vi "OLD_GUI_DO_NOT_USE-Capacitance.vi"() -> ()   [LabVIEW 2020]
uses:
  <vilib>/Utility/NIReport.llb/NI_report.lvclass
  <vilib>/Utility/NIReport.llb/Report Type.ctl
  <vilib>/addons/_office/_exclsub.llb/font.ctl
  <vilib>/addons/_office/excel.llb/Excel Easy Table (str).vi
  HP 4275A Address constant.vi
  HP 3457A Address constant.vi
  Keithley K2400 Address constant.vi
  <vilib>/Utility/NIReport.llb/NI_ReportGenerationCore.lvlib
  <vilib>/Utility/NIReport.llb/Excel/NI_Excel.lvclass
  <vilib>/addons/_office/NI_ReportGenerationToolkit.lvlib
panel:
  out "report out":refnum<class "NI_report.lvclass">
  out "error out":errorcluster
  in  "Filename":string
  in  "Test Mode":u16(ring) items=["Measure Capacitance", "Measure Series Impedance"]
  in  "function B\n(d or x/b:0)":i16(slide) scale=0.0..2.0 scale format="%.2f"
  in  "function A (c:1)":i16(slide)=1 scale=0.0..3.0 scale format="%.2f"
  out "Part Number to be Tested":u16
  in  "Number of Parts":i32
  in  "outside border":T1={"on/off"=FALSE, "weight"=2, "color"=0} {"weight" items=["xlHairline"=1, "xlMedium"=-4138, "xlThick"=4, "xlThin"=2]}
  in  "inside border":T1={"on/off"=FALSE, "weight"=2, "color"=0} {"weight" items=["xlHairline"=1, "xlMedium"=-4138, "xlThick"=4, "xlThin"=2]}
  in  "Next Part":bool
  in  "Max Voltage":dbl
  in  "Test Frequncy":string(combo)
  in  "Test System":string(combo)
  in  "Test Type":string(combo)
  in  "Date":string
  in  "Operator Name":string
  in  "Test Comments":string
  in  "Lot/Date Code":string
  in  "Lot Number":string
  in  "Request ID Number":string
  in  "Part Number":string
  in  "window state (normal)":T2(ring)=enum."normal"
  in  "FET Test Configuration":u16(ring) items=["CISS: VDS is variable, VGS=0V BLACK Jacks", "COSS: VDS is variable, a BLACK Jacks", "CRSS: VDS is variable, VGS=0V BLACK Jacks", "CISS: VDS is variable, VGS=0V RED Jacks", "COSS: VDS is variable, VGS=0V RED Jacks", "CRSS: VDS is variable, VGS=0V RED Jacks", "CIES: VDS is variable, VGS=0V Black Jacks", "CIES: VGS is variable, VDS=0V Red Jacks", "COES: VDS is variable, VGS=0V Black Jacks", "COES: VGS is variable, VDS=0V Red Jacks", "CRES: VDS is variable, VGS=0V Black Jacks", "CRES: VGS is variable, VDS=0V Red Jacks", "Special"]
  in  "Device":u16(ring) items=["Diode", "Transistor", "BRT", "MOSFET", "MOSFET with Gate Resistor", "JFET", "SSOVP", "SIDAC", "Bidirectional Zener", "SRC or TRIAC", "Darlington Transistor", "MicroIntegration", "IGBT", "IGBT with Gate Resistor", "Other"]
  in  "Transistor Test Configuration":u16(ring) items=["Cobo (Cob)", "Cibo (Cib)", "Coe", "Ccb (Cre)", "Ceb (Crc)", "Crb (Cce)", "Special"]
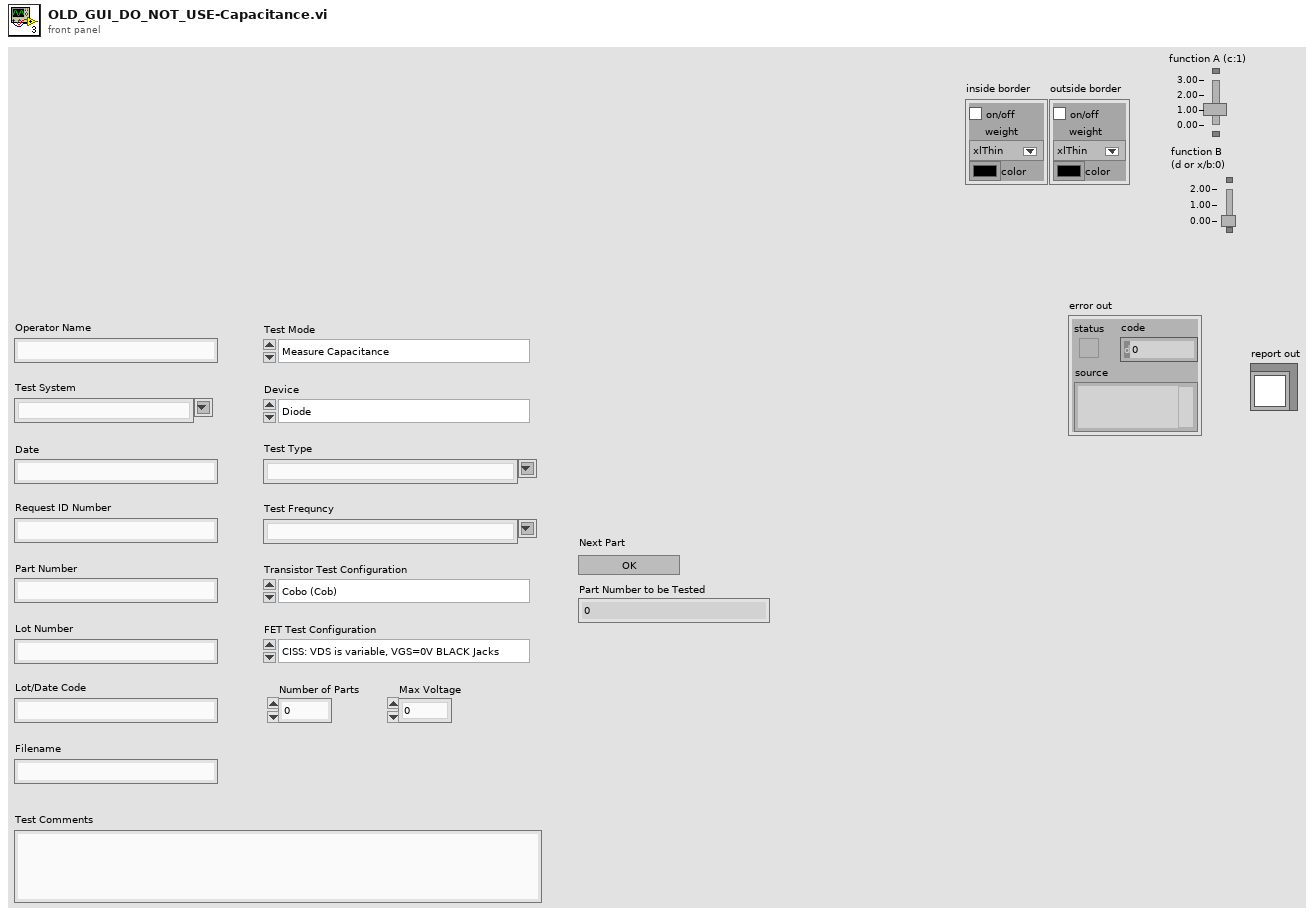
[diagram p1: front panel]
types:
  T1 = cluster{"on/off":bool, "weight":i32, "color":u32}
  T2 = enum16{"maximized", "minimized", "normal", "no change"}
  T3 = typedef "NI_ReportGenerationToolkit.lvlib/font.ctl" = cluster{"font name":string, "font size":dbl, "bold":u16, "italic":u16, "underline":u16, "strike through":u16, "font color":u32}
  T4 = typedef "NI_ReportGenerationCore.lvlib/Report Type.ctl" = enum16{"HTML", "Word", "Excel"}
  T5 = typedef "Control 1.ctl" = string
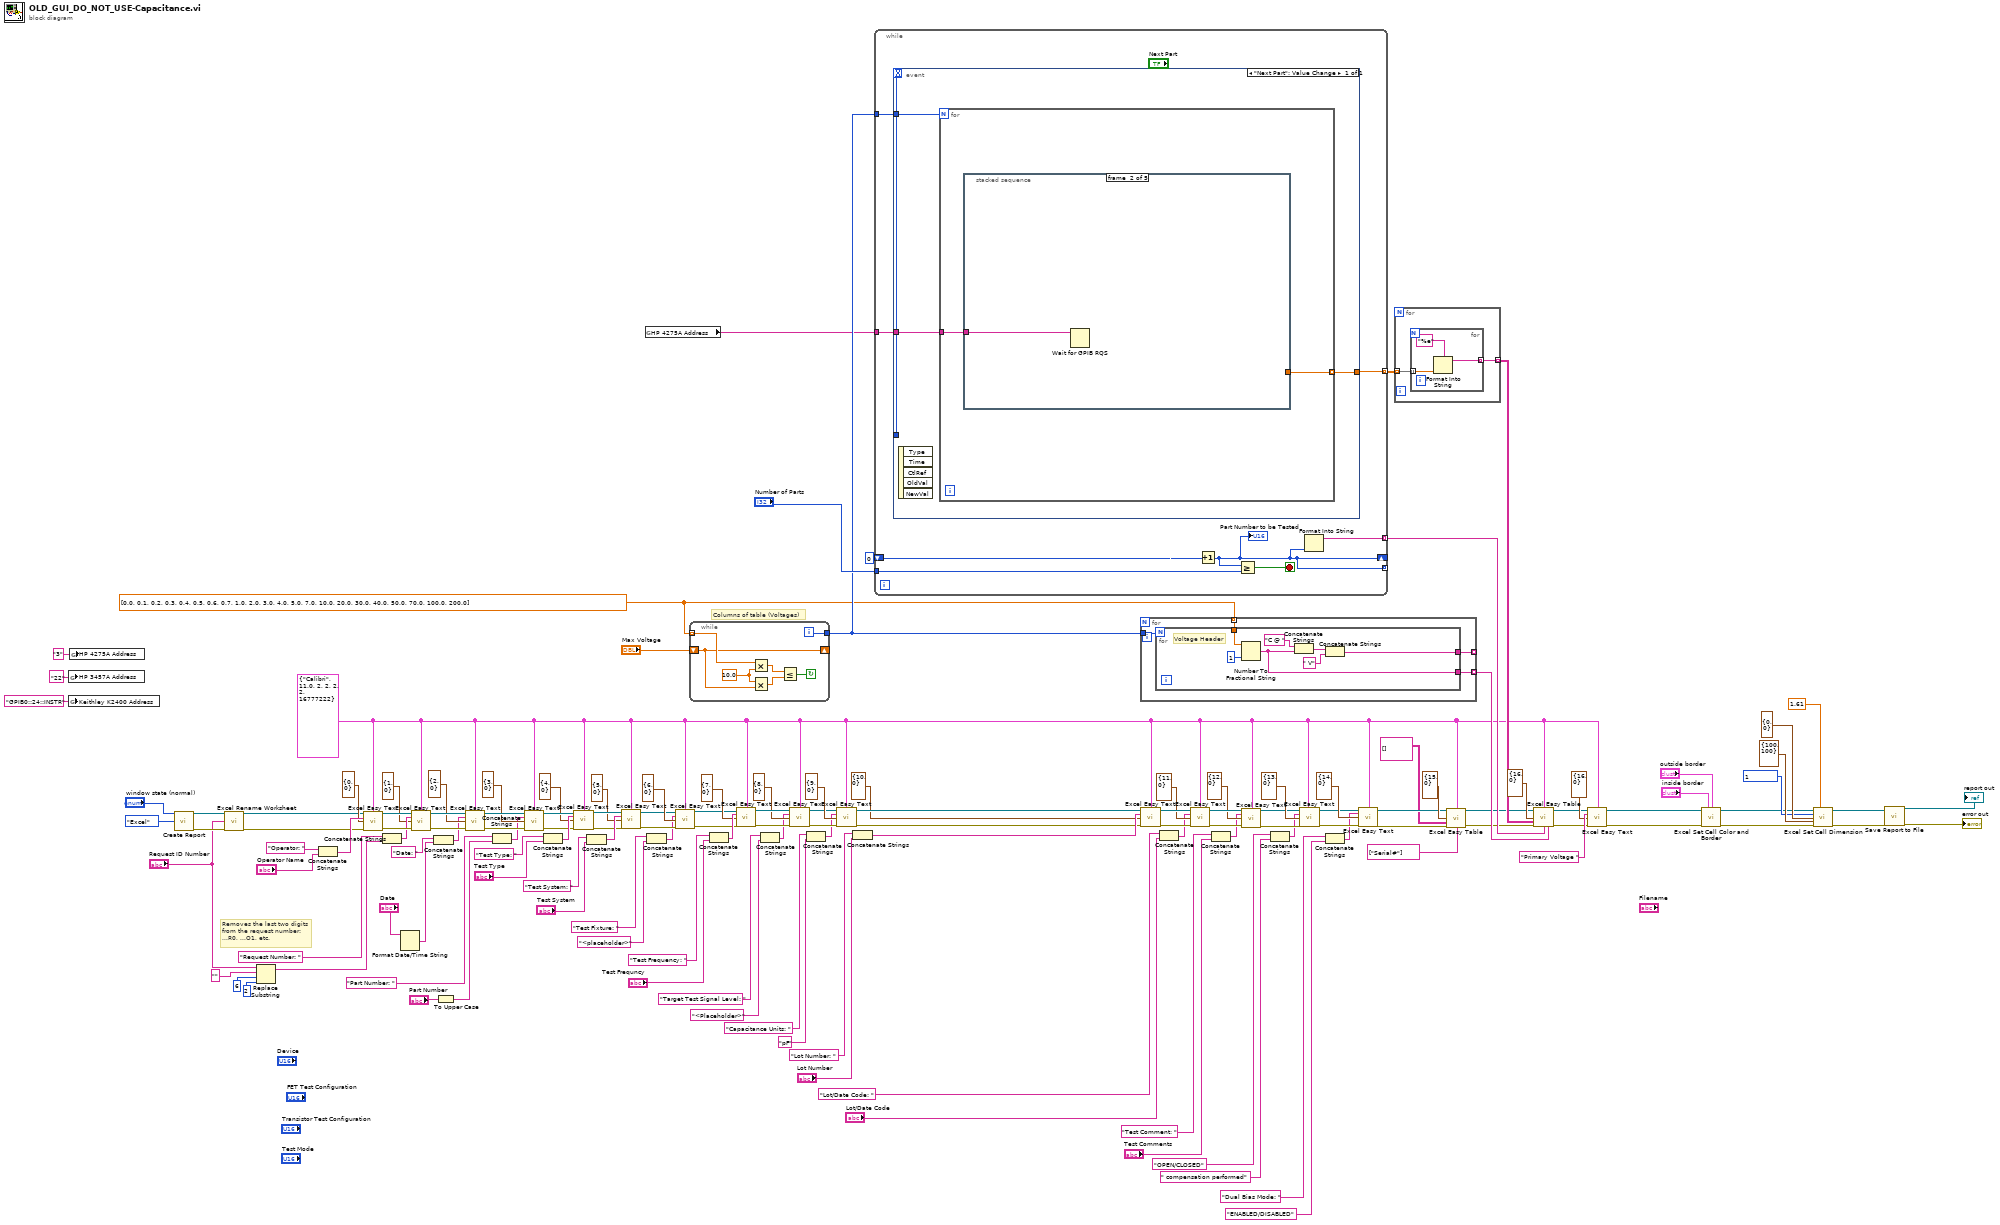
[diagram p0: block diagram]
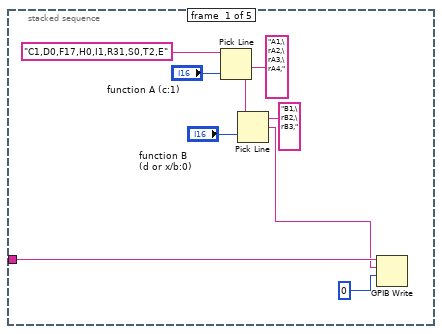
[diagram p2: hidden frame]
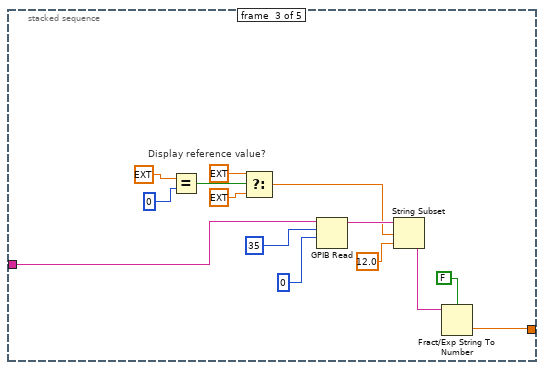
[diagram p3: hidden frame]
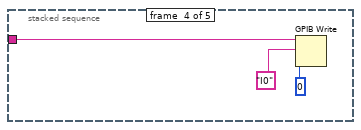
[diagram p4: hidden frame]
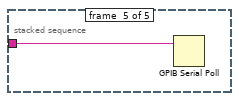
[diagram p5: hidden frame]
diagram:
  w9 = dbl[] [0.0, 0.1, 0.2, 0.3, 0.4, 0.5, 0.6, 0.7, 1.0, 2.0, 3.0, 4.0, 5.0, 7.0, 10.0, 20.0, 30.0, 40.0, 50.0, 70.0, 100.0, 200.0]
  w16 = T3 {"font name"="Calibri", "font size"=11.0, "bold"=2, "italic"=2, "underline"=2, "strike through"=2, "font color"=16777222} ("font")
  # "Columns of table (Voltages)"
  # "Removes the last two digits\nfrom the request number:\n...R0, ...O1, etc."
  n1 = global write "HP 3457A Address constant.vi" "HP 3457A Address"("22" ("HP 3457A Address")) -> ()
  n2 = global write "Keithley K2400 Address constant.vi" "Keithley K2400 Address"("GPIB0::24::INSTR" ("Keithley K2400 Address")) -> ()
  n3 = global write "HP 4275A Address constant.vi" "HP 4275A Address"("3" ("HP 4275A Address")) -> ()
  n4 = call <vilib>:"Create Report.vi"("window state (normal)"="window state (normal)", "report type"=Report_Type."Excel") -> ("report out"=w137:refnum<class "NI_report.lvclass">, "error out"=w138:errorcluster)  [unwired: 12 in]
  n5 = call <vilib>:"Excel Rename Worksheet.vi"("report in"=w137, "worksheet name (\"\")"="Request ID Number", "error in (no error)"=w138) -> ("report out"=w91:refnum<class "NI_report.lvclass">, "error out"=w92:errorcluster)  [unwired: 11 in]
  n6 = Replace Substring(2:2 ("length (len. of substring)"), 3:6 ("offset (0)"), 4:"" ("substring (\"\")"), 5:"Request ID Number") -> (1:w125:string)  [unwired: 1 out]
  n7 = Concatenate Strings("Operator: ", "Operator Name") -> (w134:string)
  n8 = call <vilib>:"Excel Easy Text.vi"("report in"=w91, "font"=w16, "text"=w134, "start (-1, -1)"=cluster{"row":i32, "column":i32} {"row"=0, "column"=0}, "error in (no error)"=w92) -> ("report out"=w132:refnum<class "NI_report.lvclass">, "error out"=w131:errorcluster)  [unwired: 6 in, 3 out]
  n9 = Concatenate Strings("Request Number: ", w125) -> (w129:string)
  n10 = Format Date/Time String(time format string (%c)="Date") -> (date/time string=w117:string)  [unwired: 2 in]
  n11 = call <vilib>:"Excel Easy Text.vi"("report in"=w132, "font"=w16, "text"=w129, "start (-1, -1)"=cluster{"row":i32, "column":i32} {"row"=1, "column"=0}, "error in (no error)"=w131) -> ("report out"=w122:refnum<class "NI_report.lvclass">, "error out"=w121:errorcluster)  [unwired: 6 in, 3 out]
  n12 = Concatenate Strings("Date: " ("string"), w117) -> (w119:string)
  n13 = To Upper Case(1:"Part Number") -> (0:w111:string)
  n14 = call <vilib>:"Excel Easy Text.vi"("report in"=w122, "font"=w16, "text"=w119, "start (-1, -1)"=cluster{"row":i32, "column":i32} {"row"=2, "column"=0}, "error in (no error)"=w121) -> ("report out"=w114:refnum<class "NI_report.lvclass">, "error out"=w113:errorcluster)  [unwired: 6 in, 3 out]
  n15 = Concatenate Strings("Part Number: " ("string"), w111) -> (w109:string)
  n16 = call <vilib>:"Excel Easy Text.vi"("report in"=w114, "font"=w16, "text"=w109, "start (-1, -1)"=cluster{"row":i32, "column":i32} {"row"=3, "column"=0}, "error in (no error)"=w113) -> ("report out"=w106:refnum<class "NI_report.lvclass">, "error out"=w105:errorcluster)  [unwired: 6 in, 3 out]
  n17 = Concatenate Strings("Test Type: " ("string"), "Test Type") -> (w107:string)
  n18 = call <vilib>:"Excel Easy Text.vi"("report in"=w106, "font"=w16, "text"=w107, "start (-1, -1)"=cluster{"row":i32, "column":i32} {"row"=4, "column"=0}, "error in (no error)"=w105) -> ("report out"=w100:refnum<class "NI_report.lvclass">, "error out"=w99:errorcluster)  [unwired: 6 in, 3 out]
  n19 = Concatenate Strings("Test System: " ("string"), "Test System") -> (w101:string)
  n20 = call <vilib>:"Excel Easy Text.vi"("report in"=w100, "font"=w16, "text"=w101, "start (-1, -1)"=cluster{"row":i32, "column":i32} {"row"=5, "column"=0}, "error in (no error)"=w99) -> ("report out"=w56:refnum<class "NI_report.lvclass">, "error out"=w55:errorcluster)  [unwired: 6 in, 3 out]
  n21 = global read "HP 4275A Address constant.vi" "HP 4275A Address"() -> (w3:T5)
  n22 = Concatenate Strings("Test Fixture: " ("string"), "<placeholder>" ("string")) -> (w52:string)
  n23 = call <vilib>:"Excel Easy Text.vi"("report in"=w56, "font"=w16, "text"=w52, "start (-1, -1)"=cluster{"row":i32, "column":i32} {"row"=6, "column"=0}, "error in (no error)"=w55) -> ("report out"=w54:refnum<class "NI_report.lvclass">, "error out"=w53:errorcluster)  [unwired: 6 in, 3 out]
  n24 = while {
    tunnel: w9 -> [w147] mode=indexing
    shift-right: [w146] -> _
    shift-left: "Max Voltage" -> [w146]
    tunnel: [w144] -> w11
    i -> [w144]
    stop <- w143 continue-if-true
    w145 = 10.0
    n25 = Multiply(x=w147, y=w145) -> (x*y=w142:dbl)
    n26 = Multiply(x=w145, y=w146) -> (x*y=w141:dbl)
    n27 = Less Or Equal?(x=w142, y=w141) -> (x <= y?=w143:bool)
  }
  n28 = Concatenate Strings("Test Frequency: " ("string"), "Test Frequncy") -> (w94:string)
  n29 = call <vilib>:"Excel Easy Text.vi"("report in"=w54, "font"=w16, "text"=w94, "start (-1, -1)"=cluster{"row":i32, "column":i32} {"row"=7, "column"=0}, "error in (no error)"=w53) -> ("report out"=w86:refnum<class "NI_report.lvclass">, "error out"=w85:errorcluster)  [unwired: 6 in, 3 out]
  n30 = Concatenate Strings("Target Test Signal Level: ", "<Placeholder>" ("string")) -> (w82:string)
  n31 = call <vilib>:"Excel Easy Text.vi"("report in"=w86, "font"=w16, "text"=w82, "start (-1, -1)"=cluster{"row":i32, "column":i32} {"row"=8, "column"=0}, "error in (no error)"=w85) -> ("report out"=w79:refnum<class "NI_report.lvclass">, "error out"=w78:errorcluster)  [unwired: 6 in, 3 out]
  n32 = Concatenate Strings("Capacitance Units: " ("string"), "pF" ("string")) -> (w77:string)
  n33 = call <vilib>:"Excel Easy Text.vi"("report in"=w79, "font"=w16, "text"=w77, "start (-1, -1)"=cluster{"row":i32, "column":i32} {"row"=9, "column"=0}, "error in (no error)"=w78) -> ("report out"=w73:refnum<class "NI_report.lvclass">, "error out"=w72:errorcluster)  [unwired: 6 in, 3 out]
  n34 = Concatenate Strings("Lot Number: " ("string"), "Lot Number") -> (w74:string)
  n35 = while {
    shift-right: [w150] -> _
    shift-left: 0 -> [w155]
    tunnel: "Number of Parts" -> [w153]
    tunnel: [w152] -> w33 mode=indexing
    tunnel: w11 -> [w151]
    tunnel: [w150] -> _ mode=indexing
    tunnel: [w149] -> w25 mode=indexing
    tunnel: w3 -> [w148]
    stop <- w154 stop-if-true
    n36 = event shown="[0] \"Next Part\": Value Change" {
      selector: _ -> [_]
      dyn-events: _ -> [_]
      timeout: _ -> [w159]
      tunnel: [w159] -> _
      tunnel: [w158] -> w152
      tunnel: w151 -> [w157]
      tunnel: w148 -> [w156]
      event "Next Part": Value Change {
        n37 = event-data() -> ()  [unwired: 1 in, 5 out]
        n38 = for {
          N: w157 -> [_]
          tunnel: [w161] -> w158 mode=indexing
          tunnel: w156 -> [w160]
          n39 = stacked-sequence {
            tunnel: [_ _ w184 _ _] -> w161
            tunnel: w160 -> [w169 w171 w183 w186 w189]
            frame #0 {
              n40 = Pick Line(string ("")="C1,D0,F17,H0,I1,R31,S0,T2,E" ("data"), multi-line string="A1,\rA2,\rA3,\rA4,", line index="function A (c:1)") -> (output string=w168:string)
              n41 = Pick Line(string ("")=w168, multi-line string="B1,\rB2,\rB3,", line index="function B\n(d or x/b:0)") -> (output string=w163:string)
              n42 = GPIB Write(0:w169, 1:w163, 2:i16 0 ("mode (0)")) -> ()  [unwired: 2 in, 2 out]
            }
            frame #1 {
              n43 = Wait for GPIB RQS(4:w171) -> ()  [unwired: 2 in, 2 out]
            }
            frame #2 {
              # "Display reference value?"
              n44 = Equal?(x=ext 3.0, y=0) -> (x = y?=w178:bool)
              n45 = Select(t=ext 3.0, s=w178, f=ext 6.0) -> (s? t:f=w174:ext)
              n46 = GPIB Read(0:w183, 1:35 ("byte count"), 2:i16 0 ("mode (0)")) -> (5:w180:string)  [unwired: 2 in, 2 out]
              n47 = String Subset(string=w180, offset (0)=w174, length (rest)=12.0) -> (substring=w179:string)
              n48 = Fract/Exp String To Number(use system decimal point (T)=FALSE, string=w179) -> (number=w184:dbl)  [unwired: 2 in, 1 out]
            }
            frame #3 {
              n49 = GPIB Write(0:w186, 1:"I0", 2:0) -> ()  [unwired: 2 in, 2 out]
            }
            frame #4 {
              n50 = GPIB Serial Poll(0:w189) -> ()  [unwired: 1 in, 3 out]
            }
          }
        }
      }
    }
    n51 = Increment(x=w155) -> (x+1=w150:i32)
    "Part Number to be Tested" <- w150
    n52 = Greater Or Equal?(x=w150, y=w153) -> (x >= y?=w154:bool)
    n53 = Format Into String(w150) -> (resulting string=w149:string)  [unwired: 3 in, 1 out]
  }
  n54 = for {
    tunnel: [w193] -> _ mode=indexing
    tunnel: w9 -> [w192] mode=indexing
    tunnel: [w190] -> w27 mode=indexing
    tunnel: w11 -> [w191]
    n55 = for {
      N: w191 -> [_]
      tunnel: w192 -> [w199]
      tunnel: [w197] -> w193
      tunnel: [w194] -> w190
      # "Voltage Header"
      n56 = Number To Fractional String(number=w199, precision (6)=i16 1) -> (F-format string=w194:string)  [unwired: 2 in]
      n57 = Concatenate Strings("C @ ", w194) -> (w196:string)
      n58 = Concatenate Strings(w196, " V" ("string")) -> (w197:string)
    }
  }
  n59 = call <vilib>:"Excel Easy Text.vi"("report in"=w73, "font"=w16, "text"=w74, "start (-1, -1)"=cluster{"row":i32, "column":i32} {"row"=10, "column"=0}, "error in (no error)"=w72) -> ("report out"=w68:refnum<class "NI_report.lvclass">, "error out"=w67:errorcluster)  [unwired: 6 in, 3 out]
  n60 = Concatenate Strings("Lot/Date Code: " ("string"), "Lot/Date Code") -> (w65:string)
  n61 = call <vilib>:"Excel Easy Text.vi"("report in"=w68, "font"=w16, "text"=w65, "start (-1, -1)"=cluster{"row":i32, "column":i32} {"row"=11, "column"=0}, "error in (no error)"=w67) -> ("report out"=w62:refnum<class "NI_report.lvclass">, "error out"=w61:errorcluster)  [unwired: 6 in, 3 out]
  n62 = Concatenate Strings("Test Comment: " ("string"), "Test Comments") -> (w59:string)
  n63 = call <vilib>:"Excel Easy Text.vi"("report in"=w62, "font"=w16, "text"=w59, "start (-1, -1)"=cluster{"row":i32, "column":i32} {"row"=12, "column"=0}, "error in (no error)"=w61) -> ("report out"=w48:refnum<class "NI_report.lvclass">, "error out"=w47:errorcluster)  [unwired: 6 in, 3 out]
  n64 = Concatenate Strings("OPEN/CLOSED" ("string"), " compensation performed" ("string")) -> (w46:string)
  n65 = call <vilib>:"Excel Easy Text.vi"("report in"=w48, "font"=w16, "text"=w46, "start (-1, -1)"=cluster{"row":i32, "column":i32} {"row"=13, "column"=0}, "error in (no error)"=w47) -> ("report out"=w42:refnum<class "NI_report.lvclass">, "error out"=w41:errorcluster)  [unwired: 6 in, 3 out]
  n66 = Concatenate Strings("Dual Bias Mode: " ("string"), "ENABLED/DISABLED" ("string")) -> (w40:string)
  n67 = call <vilib>:"Excel Easy Text.vi"("report in"=w42, "font"=w16, "text"=w40, "start (-1, -1)"=cluster{"row":i32, "column":i32} {"row"=14, "column"=0}, "error in (no error)"=w41) -> ("report out"=w13:refnum<class "NI_report.lvclass">, "error out"=w12:errorcluster)  [unwired: 6 in, 3 out]
  n68 = for {
    tunnel: w33 -> [w202] mode=indexing
    tunnel: [w201] -> w36 mode=indexing
    n69 = for {
      tunnel: w202 -> [w205] mode=indexing
      tunnel: [w204] -> w201 mode=indexing
      n70 = Format Into String(format string="%e", w205) -> (resulting string=w204:string)  [unwired: 2 in, 1 out]
    }
  }
  n71 = call-poly <vilib>:"Excel Easy Table.vi"("report in"=w13, "font"=w16, "start (0, 0)"=cluster{"row":i32, "column":i32} {"row"=15, "column"=0}, "text data"=string[][] [], "error in (no error)"=w12, "row headers"=string[] ["Serial#"]) -> ("report out"=w18:refnum<class "NI_report.lvclass">, "error out"=w17:errorcluster)  [unwired: 5 in, 3 out]
  n72 = call-poly <vilib>:"Excel Easy Table.vi"("report in"=w18, "font"=w16, "start (0, 0)"=cluster{"row":i32, "column":i32} {"row"=16, "column"=0}, "text data"=w36, "error in (no error)"=w17, "row headers"=w25, "column headers"=w27) -> ("report out"=w21:refnum<class "NI_report.lvclass">, "error out"=w22:errorcluster)  [unwired: 4 in, 3 out]
  n73 = call <vilib>:"Excel Easy Text.vi"("report in"=w21, "font"=w16, "text"="Primary Voltage ", "start (-1, -1)"=cluster{"row":i32, "column":i32} {"row"=16, "column"=0} ("start (0, 0)"), "error in (no error)"=w22) -> ("report out"=w20:refnum<class "NI_report.lvclass">, "error out"=w19:errorcluster)  [unwired: 6 in, 3 out]
  n74 = call <vilib>:"Excel Set Cell Color and Border.vi"("report in"=w20, "inside border"="inside border", "outside border"="outside border", "error in (no error)"=w19) -> ("report out"=w31:refnum<class "NI_report.lvclass">, "error out"=w32:errorcluster)  [unwired: 10 in]
  n75 = call <vilib>:"Excel Set Cell Dimension.vi"("report in"=w31, "width (-1)"=1.61, "measurement system"=u16 1, "start (-1, -1)"=cluster{"row":i32, "column":i32} {"row"=0, "column"=0}, "end (-1, -1)"=cluster{"row":i32, "column":i32} {"row"=100, "column"=100}, "error in (no error)"=w32) -> ("report out"=w5:refnum<class "NI_report.lvclass">, "error out"=w4:errorcluster)  [unwired: 8 in]
  n76 = call-dynamic "Save Report to File.vi"("report in"=w5, "error in (no error)"=w4) -> ("report out"=→"report out":refnum<class "NI_report.lvclass">, "error out"=→"error out":errorcluster)  [unwired: 12 in]
